vi "Motor test.vi"() -> ()   [LabVIEW 2011]
uses:
  <vilib>/Rock Robotics/SystemInterfaces/DIO/FPGA_DIOPWMChannel.ctl
  <vilib>/Rock Robotics/WPI/MotorControl/WPI_MotorControlOpen Jaguar.vi
panel:
  in  "stop":bool
  in  "Output":dbl(slide) scale=0.0..1.0
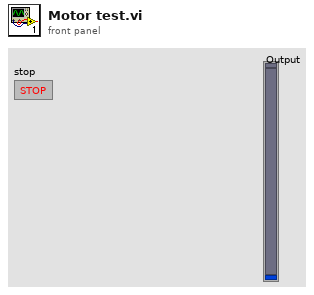
[diagram p1: front panel]
types:
  T1 = typedef "FPGA_DIOPWMChannel.ctl" = enum8{"PWM 1", "PWM 2", "PWM 3", "PWM 4", "PWM 5", "PWM 6", "PWM 7", "PWM 8", "PWM 9", "PWM 10", "Invalid"}
  T2 = typedef "WPI_MotorControlDeviceRef.ctl" = cluster{"DeviceStatus":errorcluster, "Type":enum16{"PWM", "CAN"}, "PWM":cluster{"Digital Module":T3, "PWM Channel":T1, "DeadBand":T4}, "CAN":cluster{"Device Number":u8, "Control Mode":T5, "Semaphore":T6, "Max Vout":dbl}, "Invert":bool, "TransformRef":T7, "InvTransformRef":T7}
  T3 = typedef "FPGA_TypedefDigitalModule.ctl" = enum16{"Digital Module 1", "Digital Module 2"}
  T4 = typedef "WPI_PWMDeadband.ctl" = cluster{"Name":string, "maxPositivePwm":i32, "minPositivePwm":i32, "centerPwm":i32, "maxNegativePwm":i32, "minNegativePwm":i32, "angularRange":u16}
  T5 = typedef "WPI_CANJaguar_ControlMode.ctl" = enum8{"Percent VBus", "Current", "Speed", "Position", "Voltage"}
  T6 = typedef "Semaphore RefNum" = refnum<k1>
  T7 = typedef "WPI_PWMTransform_ConPane.ctl" = refnum<vi>
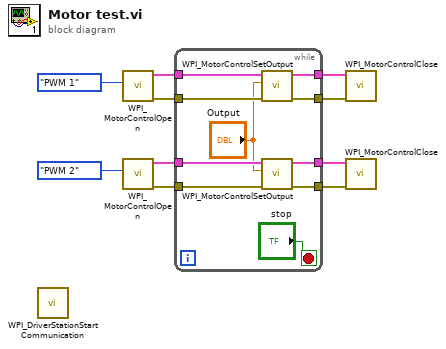
[diagram p0: block diagram]
diagram:
  n1 = call <vilib>:"WPI_DriverStationStart Communication.vi"() -> ()  [unwired: 12 in]
  n2 = call-poly <vilib>:"WPI_MotorControlOpen.vi"("PWM Channel"=FPGA_DIOPWMChannel."PWM 1") -> ("error out"=w9:errorcluster, "MotorControlDeviceRef"=w10:T2)  [unwired: 9 in]
  n3 = call-poly <vilib>:"WPI_MotorControlOpen.vi"("PWM Channel"=FPGA_DIOPWMChannel."PWM 2") -> ("error out"=w3:errorcluster, "MotorControlDeviceRef"=w4:T2)  [unwired: 9 in]
  n4 = while {
    tunnel: w10 -> [w20]
    tunnel: w9 -> [w19]
    tunnel: [w18] -> w8
    tunnel: [w17] -> w7
    tunnel: [w16] -> w6
    tunnel: [w15] -> w5
    tunnel: w4 -> [w14]
    tunnel: w3 -> [w13]
    stop <- "stop" stop-if-true
    n5 = call <vilib>:"WPI_MotorControlSetOutput.vi"("error in (no error)"=w19, "Output"="Output", "MotorControlDevRef"=w20) -> ("error out"=w17:errorcluster, "MotorControlDevRef"=w18:T2)  [unwired: 7 in]
    n6 = call <vilib>:"WPI_MotorControlSetOutput.vi"("error in (no error)"=w13, "Output"="Output", "MotorControlDevRef"=w14) -> ("error out"=w15:errorcluster, "MotorControlDevRef"=w16:T2)  [unwired: 7 in]
  }
  n7 = call <vilib>:"WPI_MotorControlClose.vi"("error in (no error)"=w7, "MotorControlDevRef"=w8) -> ()  [unwired: 9 in, 1 out]
  n8 = call <vilib>:"WPI_MotorControlClose.vi"("error in (no error)"=w5, "MotorControlDevRef"=w6) -> ()  [unwired: 9 in, 1 out]
